vi "MakePathsAbsoluteWithDefaults.vi"(8 "error in (no error)":errorcluster, 9 "relative base path":path, 10 "overrides files":path[](array[path]), 11 "system definition file":path) -> (0 "error out":errorcluster, 2 "absolute overrides files":path[](array[path]), 3 "absolute system definition file":path)   [LabVIEW 2016, in "VeriStandTestCase.lvclass"]
uses:
  VeriStandTestCase.lvclass
  <userlib>/_OpenG.lib/file/file.llb/File Exists - Scalar__ogtk.vi
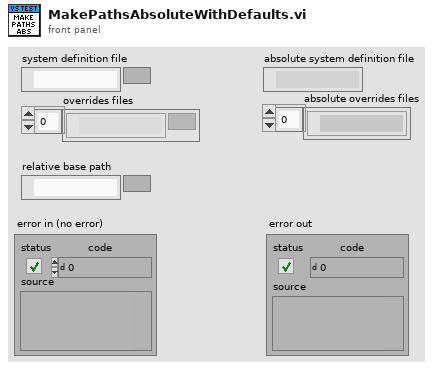
[diagram p1: front panel]
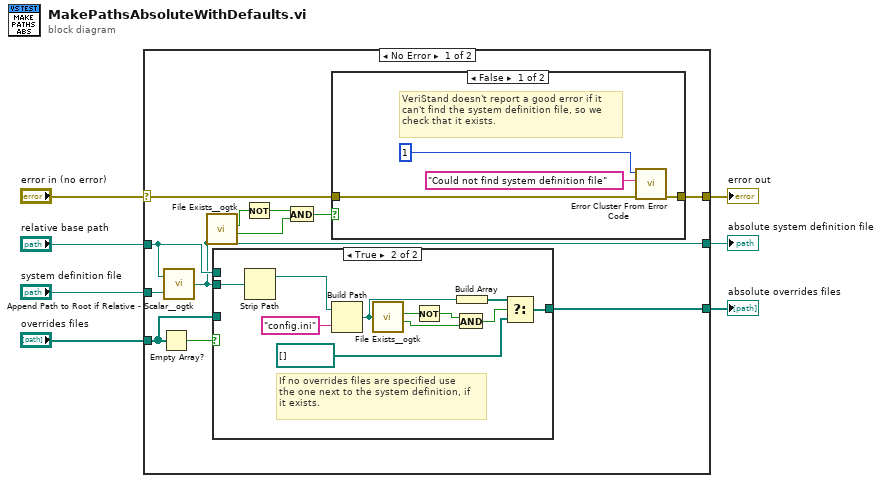
[diagram p0: block diagram]
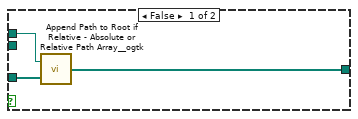
[diagram p3: hidden frame]
diagram:
  n1 = case shown="No Error" "error in (no error)" {
    selector: "error in (no error)" -> [w9 w39]
    tunnel: "overrides files" -> [w19 _]
    tunnel: [w17 _] -> w6
    tunnel: "system definition file" -> [w16 _]
    tunnel: "relative base path" -> [w15 _]
    tunnel: [w11 _] -> w3
    tunnel: [w8 w39] -> w1
    frame No Error {
      n2 = Empty Array?(array=w19) -> (empty?=w18:bool)
      n3 = call <userlib>:"Append Path to Root if Relative - Scalar__ogtk.vi"("Absolute or Relative Path"=w16, "Root Path"=w15) -> ("Absolute or Appended Path"=w11:path)
      n4 = call-poly <userlib>:"File Exists__ogtk.vi"("file path"=w11) -> ("is directory"=w14:bool, "exists"=w12:bool)  [unwired: 6 in]
      n5 = case shown="True" w18 {
        tunnel: [w27 w34] -> w17
        tunnel: w19 -> [w26 _]
        tunnel: w15 -> [w25 _]
        tunnel: w11 -> [_ w33]
        frame False {
          n6 = call <userlib>:"Append Path to Root if Relative - Absolute or Relative Path Array__ogtk.vi"("Absolute or Relative Paths"=w26, "Root Path"=w25) -> ("Absolute or Appended Paths"=w27:path[])
        }
        frame True {
          # "If no overrides files are specified use\nthe one next to the system definition, if\nit exists."
          n7 = Strip Path(path=w33) -> (stripped path=w35:path)  [unwired: 1 out]
          n8 = Build Path(base path=w35, name or relative path="config.ini") -> (appended path=w32:path)
          n9 = call-poly <userlib>:"File Exists__ogtk.vi"("file path"=w32) -> ("is directory"=w31:bool, "exists"=w29:bool)  [unwired: 6 in]
          n10 = Not(x=w31) -> (.not. x?=w30:bool)
          n11 = And(x=w30, y=w29) -> (x .and. y?=w28:bool)
          n12 = Build Array(w32) -> (w38:path[])
          n13 = Select(t=w38, s=w28, f=path[] []) -> (s? t:f=w34:path[])
        }
      }
      n14 = Not(x=w14) -> (.not. x?=w13:bool)
      n15 = And(x=w13, y=w12) -> (x .and. y?=w10:bool)
      n16 = case shown="False" w10 {
        tunnel: w9 -> [w23 w24]
        tunnel: [w22 w24] -> w8
        frame False {
          # "VeriStand doesn't report a good error if it\ncan't find the system definition file, so we\ncheck that it exists."
          n17 = call <vilib>:"Error Cluster From Error Code.vi"("error in (no error)"=w23, "error message (\"\")"="Could not find system definition file" ("error message (\"\")"), "error code (0)"=1) -> ("error out"=w22:errorcluster)  [unwired: 6 in]
        }
        frame True {
        }
      }
    }
    frame Error {
    }
  }
  "absolute overrides files" <- w6
  "absolute system definition file" <- w3
  "error out" <- w1
